vi "Configure TECs.vi"(8 "error in":errorcluster, 11 "cCRDS in":refnum<class "cCRDS.lvclass">=refnum) -> (0 "error out":errorcluster, 3 "cCRDS out":refnum<class "cCRDS.lvclass">)   [LabVIEW 2015, in "cCRDS.lvclass"]
uses:
  cCRDS.lvclass
  <vilib>/DAQmx/write.llb/DAQmx Write (Digital 1D Bool NChan 1Samp 1Line).vi
  <vilib>/DAQmx/miscellaneous.llb/DAQmx Fill In Error Info.vi
  Data Access/Write Enable.vi
  Data Access/Write AO.vi
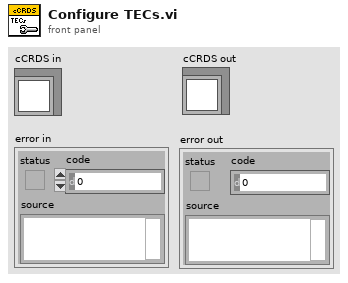
[diagram p1: front panel]
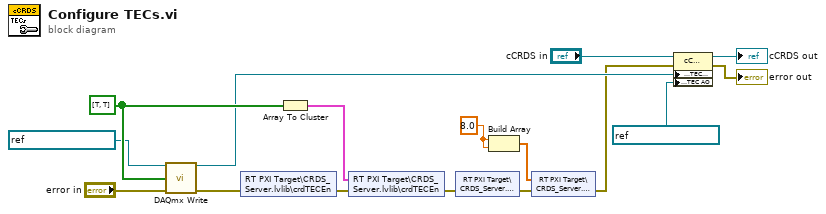
[diagram p0: block diagram]
diagram:
  w15 = sgl 8.0 ("T")
  w12 = bool[] [TRUE, TRUE] ("data")
  n1 = call-poly <vilib>:"DAQmx Write.vi"("task/channels in"=refnum<k21> "CRD Hum T En" ("Laser AI"), "data"=w12, "error in"="error in") -> ("task out"=w8:refnum<k21>, "error out"=w2:errorcluster)  [unwired: 10 in, 1 out]
  n2 = shared-variable "RT PXI Target\\CRDS_Server.lvlib\\crdTECEn"(error in=w2) -> (error out=w4:errorcluster)  [unwired: 1 out]
  n3 = Array To Cluster(array=w12) -> (cluster=w13:cluster{"data[0]":bool, "data[1]":bool})
  n4 = shared-variable "RT PXI Target\\CRDS_Server.lvlib\\crdTECEn"(w13, error in=w4) -> (error out=w5:errorcluster)
  n5 = shared-variable "RT PXI Target\\CRDS_Server.lvlib\\Tsp"(error in=w5) -> (error out=w14:errorcluster)  [unwired: 1 out]
  n6 = Build Array(w15, w15) -> (w16:sgl[])
  n7 = shared-variable "RT PXI Target\\CRDS_Server.lvlib\\Tsp"(w16, error in=w14) -> (error out=w1:errorcluster)
  n8 = property class="cCRDS"(reference="cCRDS in", error in=w1, "Accessors:TEC Enable"=w8, "Accessors:TEC AO"=refnum<k21> "CRD Hum T SP" ("TEC_AO")) -> (reference out=→"cCRDS out":refnum<class "cCRDS.lvclass">, error out=→"error out":errorcluster)
